vi "Write Simulated_CCD_Camera.lvclass.vi"(8 "error in (no error)":errorcluster, 10 "Simulated_CCD_Camera.lvclass":refnum<class "Simulated_CCD_Camera.lvclass">, 11 "Image Constructor in":refnum<class "Image Constructor.lvclass">) -> (0 "error out":errorcluster, 3 "Image Constructor out":refnum<class "Image Constructor.lvclass">)   [LabVIEW 2018, in "Image Constructor.lvclass"]
uses:
  Image Constructor.lvclass
  Simulated_CCD_Camera/Simulated_CCD_Camera.lvclass
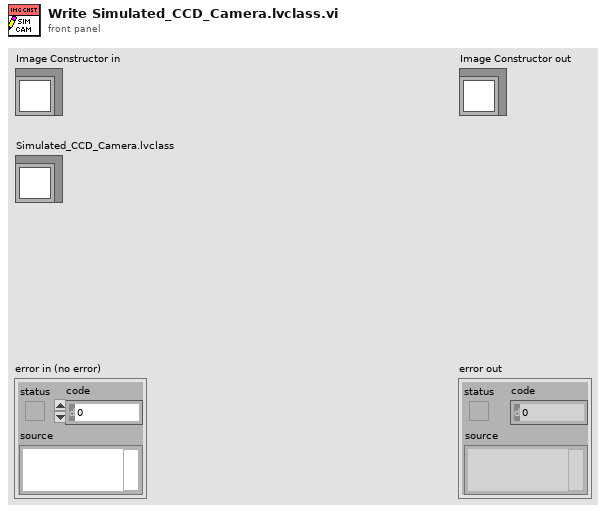
[diagram p1: front panel]
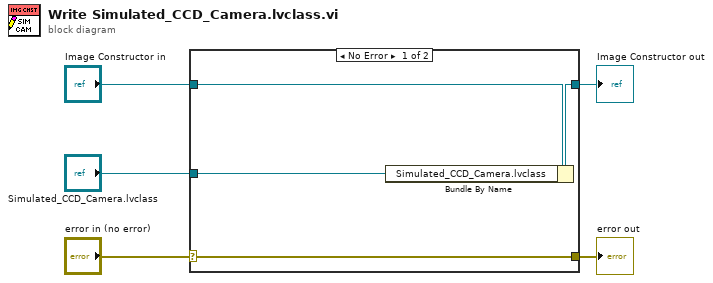
[diagram p0: block diagram]
diagram:
  n1 = case shown="No Error" "error in (no error)" {
    selector: "error in (no error)" -> [w9 w10]
    tunnel: [w9 w10] -> w4
    tunnel: [w7 w11] -> w2
    tunnel: "Image Constructor in" -> [w8 w11]
    tunnel: "Simulated_CCD_Camera.lvclass" -> [w6 _]
    frame No Error {
      n2 = Bundle By Name(cluster=w8, "Simulated_CCD_Camera.lvclass"=w6) -> (w7:refnum<class "Image Constructor.lvclass">)
    }
    frame Error {
    }
  }
  "error out" <- w4
  "Image Constructor out" <- w2
